vi "DAQ - 1-8 Modules - SubVI.vi"(11 "array":dbl[](array[numeric])) -> (3 "output array":dbl[](array[numeric]))   [LabVIEW 2013]
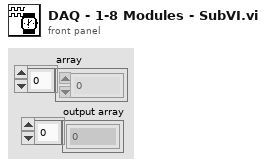
[diagram p1: front panel]
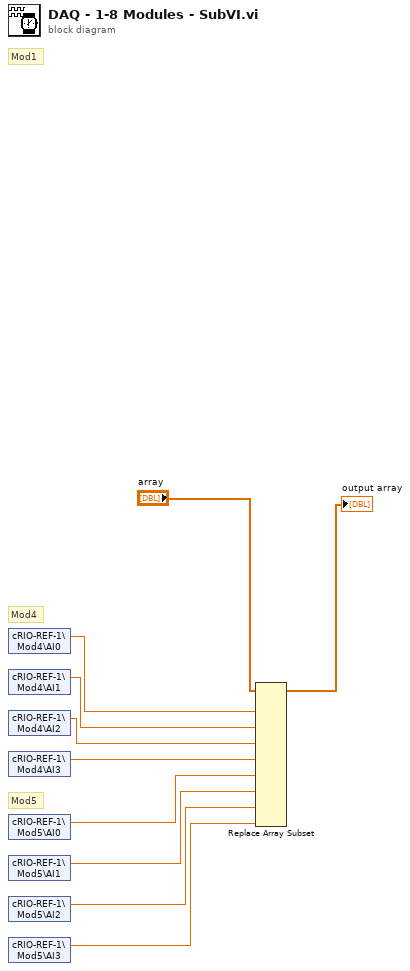
[diagram p0: block diagram]
diagram:
  # "Mod4"
  # "Mod1"
  # "Mod5"
  n1 = shared-variable "cRIO-REF-1\\Mod4\\AI0"() -> (w6:dbl)  [unwired: 1 in, 1 out]
  n2 = shared-variable "cRIO-REF-1\\Mod4\\AI1"() -> (w5:dbl)  [unwired: 1 in, 1 out]
  n3 = shared-variable "cRIO-REF-1\\Mod4\\AI2"() -> (w4:dbl)  [unwired: 1 in, 1 out]
  n4 = shared-variable "cRIO-REF-1\\Mod4\\AI3"() -> (w3:dbl)  [unwired: 1 in, 1 out]
  n5 = shared-variable "cRIO-REF-1\\Mod5\\AI0"() -> (w10:dbl)  [unwired: 1 in, 1 out]
  n6 = shared-variable "cRIO-REF-1\\Mod5\\AI1"() -> (w9:dbl)  [unwired: 1 in, 1 out]
  n7 = shared-variable "cRIO-REF-1\\Mod5\\AI2"() -> (w8:dbl)  [unwired: 1 in, 1 out]
  n8 = shared-variable "cRIO-REF-1\\Mod5\\AI3"() -> (w7:dbl)  [unwired: 1 in, 1 out]
  n9 = Replace Array Subset(array="array", new element #1=w6, new element #2=w5, new element #3=w4, new element #4=w3, new element #5=w10, new element #6=w9, new element #7=w8, new element #8=w7) -> (→"output array":dbl[])  [unwired: 8 in]
